vi "InsertOneRecordToLast2DListCtrl.vi"(10 "arr data":string[](array[string]), 11 "testcaselist in":refnum<vi>) -> (3 "testcaselist out":refnum<vi>)   [LabVIEW 2018, in "Library-Ctrl.lvlib"]
uses:
  Library-Ctrl.lvlib
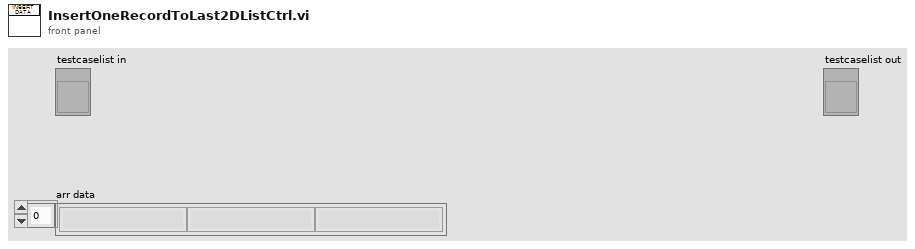
[diagram p1: front panel]
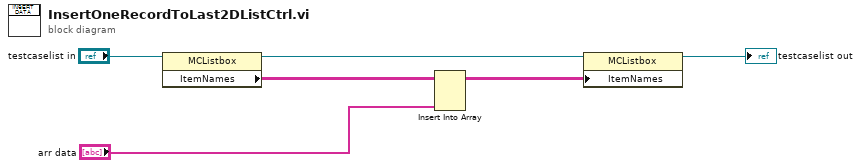
[diagram p0: block diagram]
diagram:
  n1 = property class="MCListbox"(reference="testcaselist in") -> (reference out=w4:refnum<vi>, "ItemNames"=w3:string[][])  [unwired: 1 in, 1 out]
  n2 = Insert Into Array(array=w3, new element="arr data") -> (w1:string[][])  [unwired: 2 in]
  n3 = property class="MCListbox"(reference=w4, "ItemNames"=w1) -> (reference out=→"testcaselist out":refnum<vi>)  [unwired: 1 in, 1 out]
